vi "Eval Condition.vi"(7 "Variables":refnum<class "Variables.lvclass">, 8 "error in (no error)":errorcluster, 9 "Sequence Time":T1, 11 "LowLimit Condition in":refnum<class "LowLimit Condition.lvclass">) -> (0 "error out":errorcluster, 2 "Result":bool, 3 "LowLimit Condition out":refnum<class "LowLimit Condition.lvclass">)   [LabVIEW 2020, in "VolatusSeq.lvlib" / "LowLimit Condition.lvclass"]
uses:
  LowLimit Condition.lvclass
  Sequence Time.ctl
  Variables/Variables.lvclass
  LowLimit Condition.lvclass/LowLimit Condition.ctl
  lv-vecto/Vecto/Channel DBL/Channel DBL.lvclass/Channel DBL.ctl
  lv-vecto/Vecto/Group DBL/Value by Index.vi
  Condition Value/Condition Value.lvclass
  VolatusSeq.lvlib
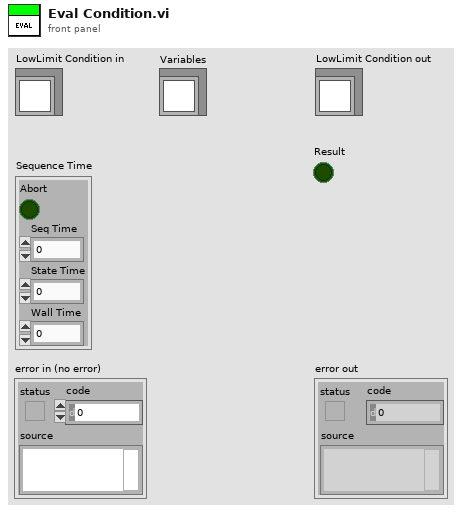
[diagram p1: front panel]
types:
  T1 = typedef "VolatusSeq.lvlib/Sequence Time.ctl" = cluster{"Abort":bool, "Seq Time":dbl, "State Time":dbl, "Wall Time":dbl}
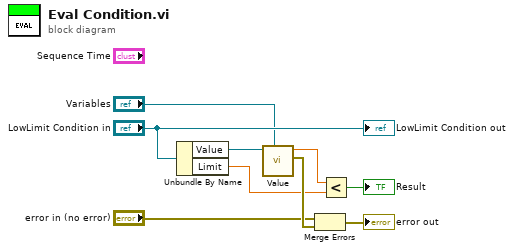
[diagram p0: block diagram]
diagram:
  n1 = Unbundle By Name("LowLimit Condition in") -> ("Value"=w6:refnum<class "Condition Value.lvclass">, "Limit"=w4:dbl)
  n2 = call "Value.vi"("Variables"="Variables", "Condition Value in"=w6) -> ("error out"=w9:errorcluster, "Value"=w5:dbl)  [unwired: 8 in]
  n3 = Merge Errors("error in (no error)", w9) -> (→"error out":errorcluster)
  n4 = Less?(x=w5, y=w4) -> (x < y?=→"Result":bool)
  "LowLimit Condition out" <- "LowLimit Condition in"
